vi "CreateNewProgect.vi"(1 "selected path":path) -> (0 "Boolean":bool)   [LabVIEW 2010]
uses:
  <vilib>/Utility/sysdir.llb/System Directory Type.ctl
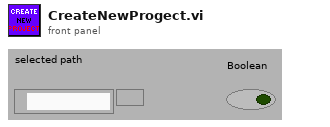
[diagram p1: front panel]
types:
  T1 = typedef "System Directory Type.ctl" = i32
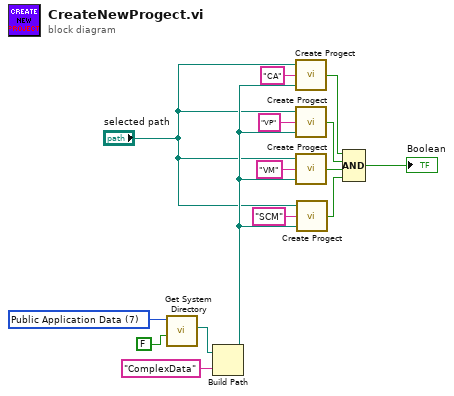
[diagram p0: block diagram]
diagram:
  w6 = T1 7 items=["User Home"=0, "User Desktop"=1, "User Documents"=2, "User Application Data"=3, "User Preferences"=4, "User Temporary"=5, "Public Documents"=6, "Public Application Data"=7, "Public Preferences"=8, "Public Cache"=13, "System Core Libraries"=9, "System Installed Libraries"=10, "Application Files"=11, "Boot Volume Root"=12] ("system directory type")
  n1 = call <vilib>:"Get System Directory.vi"("create directory if not found? (F)"=FALSE, "system directory type"=w6) -> ("system directory"=w4:path)  [unwired: 9 in]
  n2 = Build Path(base path=w4, name or relative path="ComplexData") -> (appended path=w2:path)
  n3 = call "Create Progect.vi"("Source DIR"=w2, "element"="CA", "selected path"="selected path") -> ("Boolean"=w11:bool)
  n4 = call "Create Progect.vi"("Source DIR"=w2, "element"="VP", "selected path"="selected path") -> ("Boolean"=w12:bool)
  n5 = call "Create Progect.vi"("Source DIR"=w2, "element"="VM", "selected path"="selected path") -> ("Boolean"=w14:bool)
  n6 = call "Create Progect.vi"("Source DIR"=w2, "element"="SCM", "selected path"="selected path") -> ("Boolean"=w13:bool)
  n7 = Compound Arithmetic op=AND(w11, w12, w14, w13) -> (→"Boolean":bool)
